vi "Data_Decimate - Copie.vi"(8 "error in (no error)":errorcluster, 10 "Dataset":cluster{sgl[], sgl[]}[](array[cluster]), 11 "GraphXY":refnum<vi>) -> (0 "error out":errorcluster)   [LabVIEW 2015]
doc: "This VI is a standalone test for the PXIe-5122 digitizer.\n\nIf software trigger is used, the acquisition starts immediately reading channel 0.\nIf an external trigger is used, please connect a TTL trigger to the EXT TRIG connector in front panel of the PXIe-5122 board."
uses:
  Global_Variables.vi
panel:
  out "Number of Points Currently Displayed":i32
  out "Decimation Factor":u32
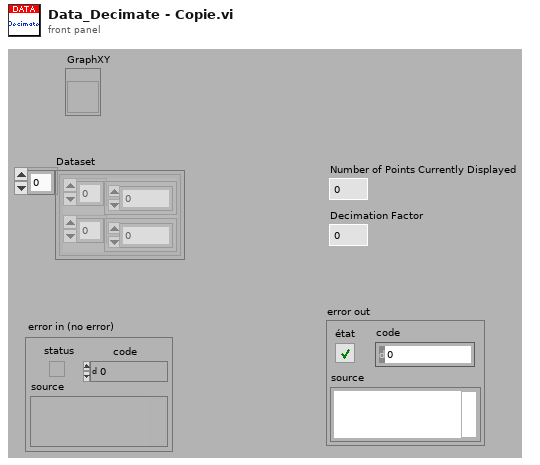
[diagram p1: front panel]
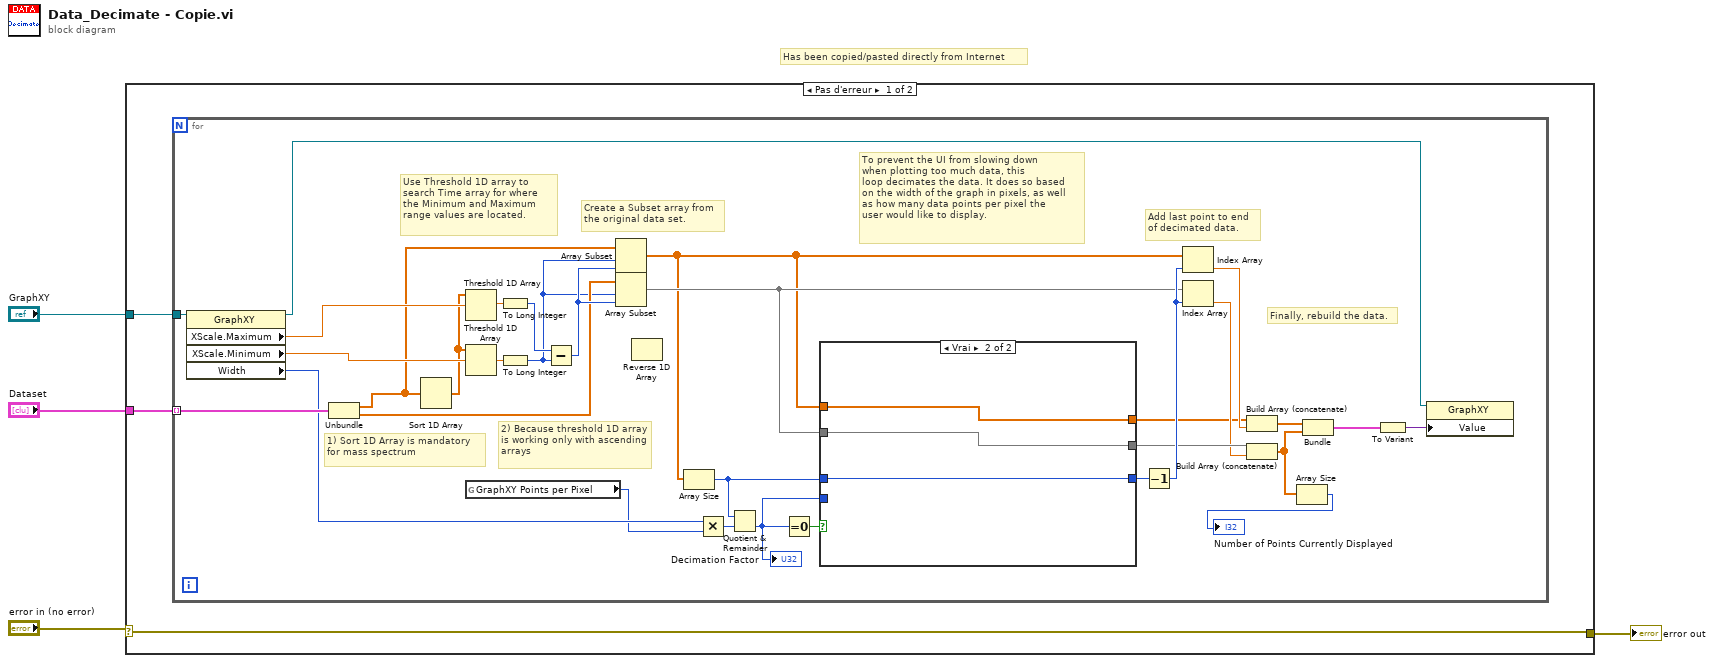
[diagram p0: block diagram]
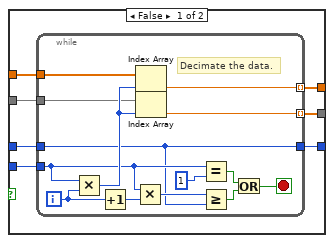
[diagram p2: hidden frame]
diagram:
  # "Has been copied/pasted directly from Internet"
  n1 = case shown="Pas d'erreur" "error in (no error)" {
    selector: "error in (no error)" -> [w5 w64]
    tunnel: [w5 w64] -> w3
    tunnel: "GraphXY" -> [w6 _]
    tunnel: "Dataset" -> [w7 _]
    frame No Error {
      n2 = for {
        tunnel: w7 -> [w39] mode=indexing
        tunnel: w6 -> [w38]
        # "1) Sort 1D Array is mandatory for mass spectrum"
        # "2) Because threshold 1D array is working only with ascending arrays"
        # "Add last point to end\nof decimated data."
        # "Finally, rebuild the data."
        # "To prevent the UI from slowing down\nwhen plotting too much data, this\nloop decimates the data. It does so based\non the width of the graph in pixels, as well\nas how many data points per pixel the\nuser would like to display."
        # "Create a Subset array from\nthe original data set."
        # "Use Threshold 1D array to\nsearch Time array for where\nthe Minimum and Maximum\nrange values are located."
        n3 = property class="GraphXY"(reference=w38) -> (reference out=w11:refnum<vi>, "XScale.Maximum"=w17:dbl, "XScale.Minimum"=w16:dbl, "Width"=w13:u32)  [unwired: 1 in, 1 out]
        n4 = Unbundle(w39) -> (w8:sgl[], w35:sgl[])
        n5 = Sort 1D Array(array=w8) -> (sorted array=w9:sgl[])
        n6 = Threshold 1D Array(2:w17, 3:w9) -> (0:w34:sgl)  [unwired: 1 in]
        n7 = Threshold 1D Array(2:w16, 3:w9) -> (0:w33:sgl)  [unwired: 1 in]
        n8 = global read "Global_Variables.vi" "GraphXY Points per Pixel"() -> (w10:i32)
        n9 = To Long Integer(number=w34) -> (32bit integer=w25:i32)
        n10 = To Long Integer(number=w33) -> (32bit integer=w24:i32)
        n11 = Subtract(x=w25, y=w24) -> (x-y=w36:i32)
        n12 = Array Subset(array=w8, index=w24, length=w36) -> (w19:sgl[])
        n13 = Array Subset(array=w35, index=w24, length=w36) -> (w30:sgl[])
        n14 = Reverse 1D Array() -> ()  [unwired: 1 in, 1 out]
        n15 = Array Size(array=w19) -> (size(s)=w23:i32)
        n16 = Multiply(x=w13, y=w10) -> (x*y=w20:u32)
        n17 = Quotient & Remainder(x=w23, y=w20) -> (floor(x/y)=w18:u32)  [unwired: 1 out]
        "Decimation Factor" <- w18
        n18 = Equal To 0?(x=w18) -> (x = 0?=w21:bool)
        n19 = case shown="Vrai" w21 {
          tunnel: [w46 w61] -> w32
          tunnel: w19 -> [w45 w63]
          tunnel: w30 -> [w44 w62]
          tunnel: [w43 w62] -> w29
          tunnel: w23 -> [w42 w61]
          tunnel: [w41 w63] -> w22
          tunnel: w18 -> [w40 _]
          frame False {
            n20 = while {
              tunnel: w45 -> [w57]
              tunnel: w44 -> [w53]
              tunnel: w42 -> [w50]
              tunnel: [w55] -> w41 mode=indexing
              tunnel: [w54] -> w43 mode=indexing
              tunnel: w40 -> [w52]
              tunnel: [w50] -> w46
              i -> [w60]
              stop <- w49 stop-if-true
              # "Decimate the data."
              n21 = Multiply(x=w52, y=w60) -> (x*y=w56:u32)
              n22 = Increment(x=w60) -> (x+1=w59:i32)
              n23 = Multiply(x=w52, y=w59) -> (x*y=w58:u32)
              n24 = Index Array(array=w57, index=w56) -> (element=w55:sgl)
              n25 = Index Array(array=w53, index=w56) -> (element=w54:sgl)
              n26 = Equal?(x=w52, y=u32 1) -> (x = y?=w48:bool)
              n27 = Greater Or Equal?(x=w58, y=w50) -> (x >= y?=w47:bool)
              n28 = Or(x=w48, y=w47) -> (x .or. y?=w49:bool)
            }
          }
          frame True {
          }
        }
        n29 = Decrement(x=w32) -> (x-1=w31:i32)
        n30 = Index Array(array=w19, index=w31) -> (element=w26:sgl)
        n31 = Index Array(array=w30, index=w31) -> (element=w28:sgl)
        n32 = Build Array (concatenate)(w22, w26) -> (w27:sgl[])
        n33 = Build Array (concatenate)(w29, w28) -> (w12:sgl[])
        n34 = Array Size(array=w12) -> (size(s)=→"Number of Points Currently Displayed":i32)
        n35 = Bundle(w27, w12) -> (w14:cluster{sgl[], sgl[]})  [unwired: 1 in]
        n36 = To Variant(anything=w14) -> (Variant=w15:variant)
        n37 = property class="GraphXY"(reference=w11, "Value"=w15) -> ()  [unwired: 1 in, 2 out]
      }
    }
    frame Error {
    }
  }
  "error out" <- w3
